vi "host_command_list.vi"() -> (2 "paths":path[](array[path]), 3 "names":string[](array[string]))   [LabVIEW 2021]
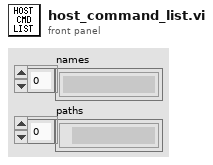
[diagram p1: front panel]
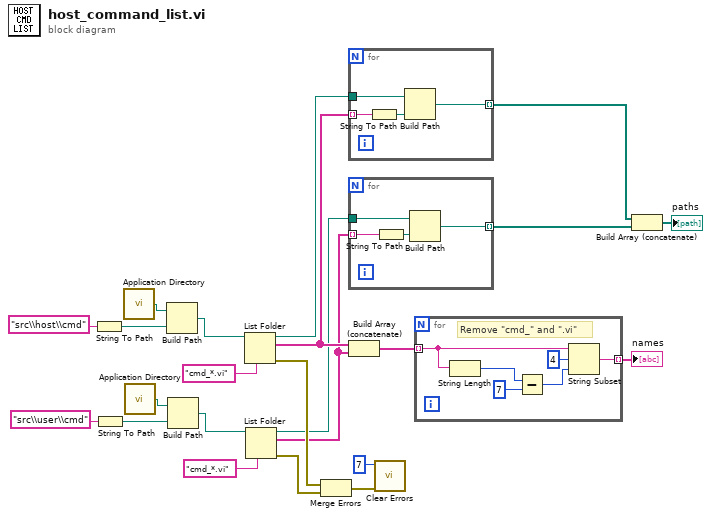
[diagram p0: block diagram]
diagram:
  n1 = String To Path(string="src\\host\\cmd") -> (path=w21:path)
  n2 = String To Path(string="src\\user\\cmd") -> (path=w16:path)
  n3 = call <vilib>:"Application Directory.vi"() -> ("Application Directory"=w23:path)
  n4 = call <vilib>:"Application Directory.vi"() -> ("Application Directory"=w14:path)
  n5 = Build Path(base path=w23, name or relative path=w21) -> (appended path=w20:path)
  n6 = Build Path(base path=w14, name or relative path=w16) -> (appended path=w17:path)
  n7 = List Folder(path=w20, pattern="cmd_*.vi") -> (path out=w7:path, filenames=w6:string[], error out=w11:errorcluster)  [unwired: 2 in, 1 out]
  n8 = List Folder(path=w17, pattern="cmd_*.vi") -> (path out=w5:path, filenames=w4:string[], error out=w10:errorcluster)  [unwired: 2 in, 1 out]
  n9 = Merge Errors(w11, w10) -> (w9:errorcluster)
  n10 = for {
    tunnel: w7 -> [w27]
    tunnel: w6 -> [w25] mode=indexing
    tunnel: [w24] -> w3 mode=indexing
    n11 = String To Path(string=w25) -> (path=w26:path)
    n12 = Build Path(base path=w27, name or relative path=w26) -> (appended path=w24:path)
  }
  n13 = for {
    tunnel: w5 -> [w30]
    tunnel: w4 -> [w29] mode=indexing
    tunnel: [w28] -> w2 mode=indexing
    n14 = String To Path(string=w29) -> (path=w31:path)
    n15 = Build Path(base path=w30, name or relative path=w31) -> (appended path=w28:path)
  }
  n16 = Build Array (concatenate)(w6, w4) -> (w13:string[])
  n17 = call <vilib>:"Clear Errors.vi"("error in (no error)"=w9, "specific error code to clear (0: all)"=7) -> ()  [unwired: 4 in, 2 out]
  n18 = for {
    tunnel: w13 -> [w33] mode=indexing
    tunnel: [w32] -> w12 mode=indexing
    # "Remove \"cmd_\" and \".vi\""
    n19 = String Length(string=w33) -> (length=w35:i32)
    n20 = Subtract(x=w35, y=7) -> (x-y=w36:i32)
    n21 = String Subset(string=w33, offset (0)=4, length (rest)=w36) -> (substring=w32:string)
  }
  "names" <- w12
  n22 = Build Array (concatenate)(w3, w2) -> (→"paths":path[])
